vi "TDV_WriteJsonMetadata.vi"(8 "error in (no error)":errorcluster, 10 "Metadata Cluster":T1, 11 "JSON destination":path) -> (0 "error out":errorcluster, 1 "JSON Refnum Out":refnum<file>, 2 "JSON String":string, 3 "JSON Destination Out":path)   [LabVIEW 2016]
uses:
  METADATA.ctl
  <vilib>/addons/_JKI.lib/Serialization/JSON/JKI JSON Serialization.lvlib
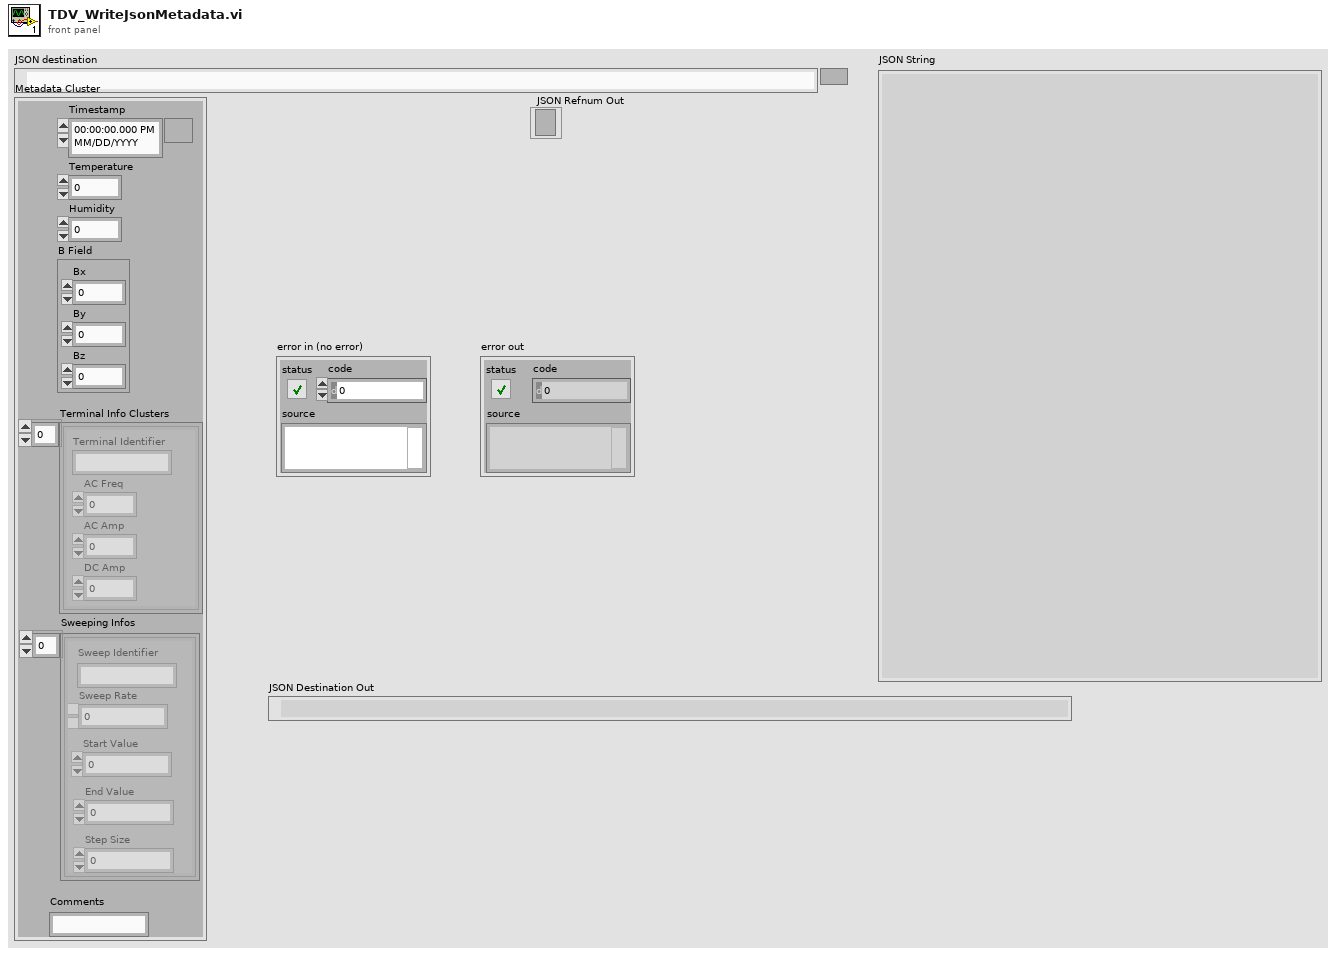
[diagram p1: front panel]
types:
  T1 = typedef "METADATA.ctl" = cluster{"Timestamp":timestamp, "Temperature":dbl, "Humidity":dbl, "B Field":cluster{"Bx":dbl, "By":dbl, "Bz":dbl}, "Terminal Info Clusters":cluster{"Terminal Identifier":string, "AC Freq":dbl, "AC Amp":dbl, "DC Amp":dbl}[], "Sweeping Infos":cluster{"Sweep Rate":dbl, "Sweep Identifier":string, "Start Value":dbl, "End Value":dbl, "Step Size":dbl}[], "Comments":string}
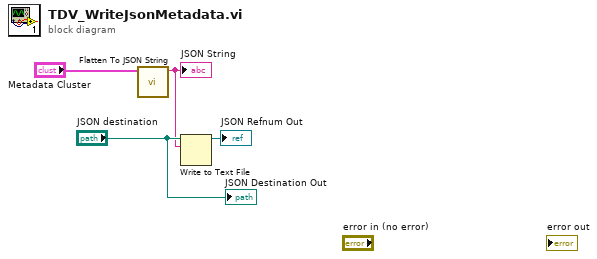
[diagram p0: block diagram]
diagram:
  n1 = call <vilib>:"Flatten To JSON String.vi"("Variant"="Metadata Cluster") -> ("JSON String"=w2:string)  [unwired: 9 in, 1 out]
  "JSON String" <- w2
  n2 = Write to Text File(file (use dialog)="JSON destination", text=w2) -> (refnum out=→"JSON Refnum Out":refnum<file>)  [unwired: 2 in, 2 out]
  "JSON Destination Out" <- "JSON destination"
